vi "parse ring controls v1_0_0.vi"(8 "error in":errorcluster, 11 "data":variant[][](array[variant])) -> (0 "error out":errorcluster, 3 "Array":string[][](array[string]))   [LabVIEW 2009]
doc: "parse ring control v1_0_0.vi\n\nthis is a cleaned and modified version of code found in the NI database connectivity toolset. It has been modified to be used as a general conversion from a Varient data type to a 2D string array/\n\ncreated 2002\nBy J. Daren Suntych\nNational Analytics\n970-397-0764"
uses:
  <vilib>/addons/database/_DB Variant To Data/Database Variant To Data.xnode
panel:
  out "subarray":variant[](array[variant])
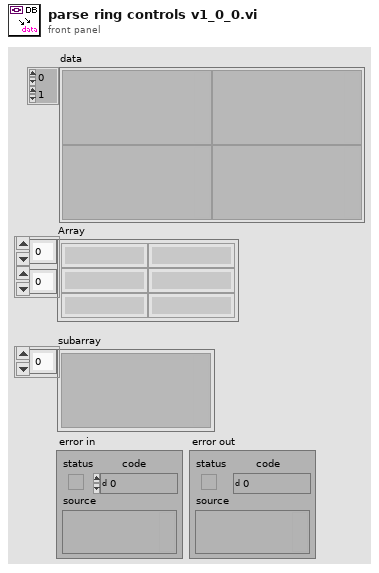
[diagram p1: front panel]
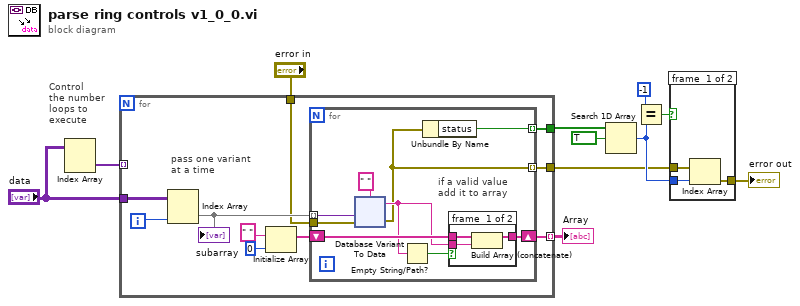
[diagram p0: block diagram]
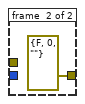
[diagram p2: hidden frame]
diagram:
  # "Control\nthe number\nloops to\nexecute"
  n1 = Index Array(array="data") -> (element=w11:variant[])  [unwired: 2 in]
  n2 = for {
    tunnel: "data" -> [w21]
    tunnel: w11 -> [_] mode=indexing
    tunnel: [w19] -> w9 mode=indexing
    tunnel: "error in" -> [w14]
    tunnel: [w13] -> w2
    tunnel: [w12] -> w4
    i -> [w20]
    # "pass one variant \nat a time"
    n3 = Index Array(array=w21, index (col)=w20) -> (element=w17:variant[])  [unwired: 1 in]
    "subarray" <- w17
    n4 = Initialize Array(" ", 0 ("dimension size")) -> (w15:string[])
    n5 = for {
      tunnel: w17 -> [w29] mode=indexing
      shift-right: [w28] -> w19
      shift-left: w15 -> [w27]
      tunnel: w14 -> [w24]
      tunnel: [w23] -> w13 mode=indexing
      tunnel: [w22] -> w12 mode=indexing
      # "if a valid value\nadd it to array"
      n6 = xnode "Database Variant To Data"("database variant"=w29, "error in"=w24, "type"=" ") -> ("data"=w26:string, "error out"=w23:errorcluster)
      n7 = Empty String/Path?(string/path=w26) -> (empty?=w25:bool)
      n8 = Unbundle By Name(w23) -> ("status"=w22:bool)
      n9 = case shown="False" w25 {
        tunnel: [w65 w66] -> w28
        tunnel: w27 -> [w64 w66]
        tunnel: w26 -> [w63 _]
        frame #0 {
          n10 = Build Array (concatenate)(w64, w63) -> (w65:string[])
        }
        frame #1 {
        }
      }
    }
  }
  "Array" <- w9
  n11 = Search 1D Array(1D array=w4, element=TRUE ("status")) -> (index of element=w5:i32)  [unwired: 1 in]
  n12 = Equal?(x=-1, y=w5) -> (x = y?=w6:bool)
  n13 = case shown="False" w6 {
    tunnel: w5 -> [w69 _]
    tunnel: w2 -> [w68 _]
    tunnel: [w67 errorcluster {"status"=FALSE, "code"=0, "source"=""} ("error out")] -> w1
    frame #0 {
      n14 = Index Array(array=w68, index=w69) -> (element=w67:errorcluster)
    }
    frame #1 {
    }
  }
  "error out" <- w1
